vi "UDP Refresh Specific Channel and Tags.vi"(8 "error in (no error)":errorcluster, 11 "node References":T1) -> (0 "error out":errorcluster, 1 "Mapped Tag Name":string, 2 "Channel Exists?":bool, 3 "node References out":T1, 4 "tags available for mapping":refnum<class "tag descriptor.lvclass">[](array[class]))   [LabVIEW 2015, in "E2E Tag Exchange editor node.lvclass"]
uses:
  E2E Tag Exchange editor node.lvclass
  object references.ctl
  <vilib>/NI/DCAF/Tag Editor Core/Configuration Editor/Classes/Engine Parent/Engine Parent Editor Node.lvclass
  <vilib>/NI/Tag Bus/tag/tag descriptor.lvclass
  <vilib>/NI/Tag Bus Module Framework/channel/TBM channel.lvclass
  <vilib>/NI/Tag Bus/tag/tag descriptor.lvclass/tag descriptor.ctl
  <vilib>/NI/Module Execution Interface/Engine Configuration/engine configuration.lvclass
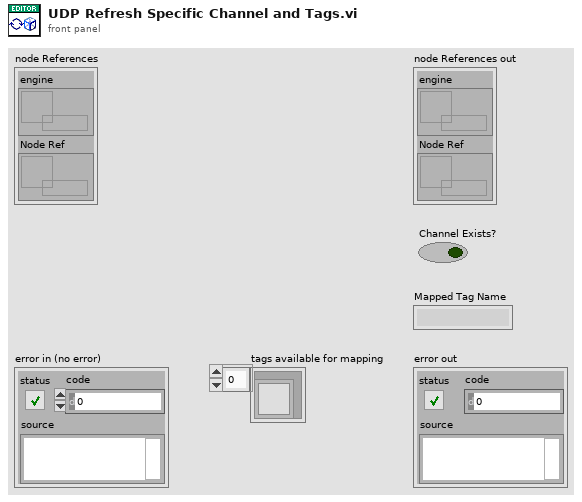
[diagram p1: front panel]
types:
  T1 = typedef "E2E Tag Exchange editor node.lvclass/object references.ctl" = cluster{"engine":refnum<data-value>, "Node Ref":refnum<data-value>}
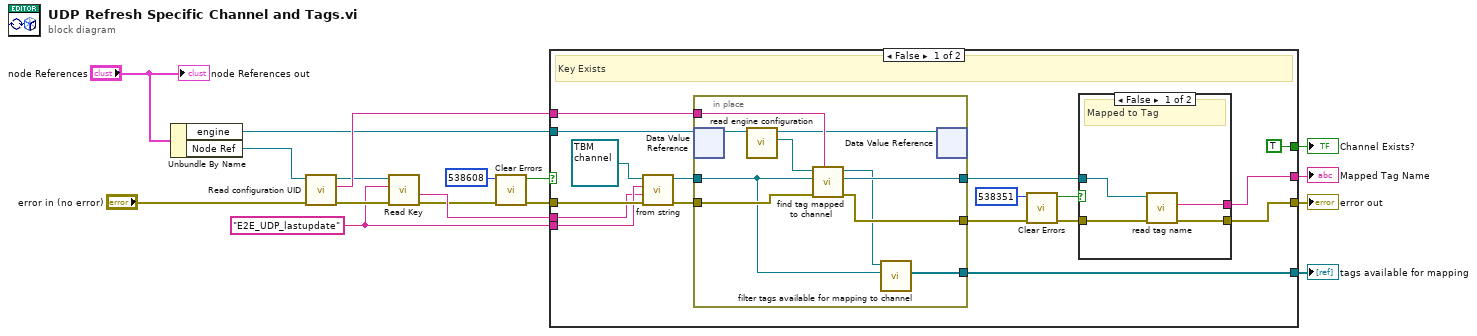
[diagram p0: block diagram]
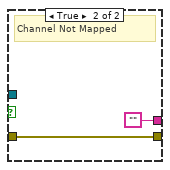
[diagram p2: hidden frame]
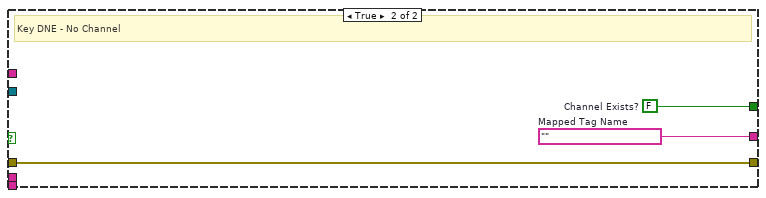
[diagram p3: hidden frame]
diagram:
  w8 = "E2E_UDP_lastupdate" ("Key")
  n1 = Unbundle By Name("node References") -> ("engine"=w10:refnum<data-value>, "Node Ref"=w14:refnum<data-value>)
  n2 = call "Read configuration UID.vi"("error in (no error)"="error in (no error)", "E2E editor node in"=w14) -> ("error out"=w12:errorcluster, "Module UID"=w13:string, "E2E editor node out"=w11:refnum<data-value>)  [unwired: 7 in]
  n3 = call "Read Key.vi"("error in (no error)"=w12, "Key"=w8, "E2E editor node in"=w11) -> ("error out"=w4:errorcluster, "Value"=w9:string)  [unwired: 6 in, 1 out]
  n4 = call <vilib>:"Clear Errors.vi"("error in (no error)"=w4, "specific error code to clear (0: all)"=538608 ("error code (0)")) -> ("error out"=w7:errorcluster, "specific error cleared?"=w6:bool)  [unwired: 4 in]
  n5 = case shown="False" w6 {
    tunnel: w7 -> [w34 w53]
    tunnel: w8 -> [w33 _]
    tunnel: w9 -> [w32 _]
    tunnel: w10 -> [w30 _]
    tunnel: w13 -> [w29 _]
    tunnel: [w21 w53] -> w2
    tunnel: [w20 w52] -> w16
    tunnel: [TRUE ("Channel Exists?") w51] -> w15
    tunnel: [w18 _] -> w1
    frame False {
      # "Key Exists"
      n6 = call-dynamic "from string.vi"("error in"=w34, "channel data"=w32, "identifier"=w33, "channel in"=refnum<class "TBM channel.lvclass"> refnum) -> ("error out"=w27:errorcluster, "channel out"=w28:refnum<class "TBM channel.lvclass">)  [unwired: 6 in]
      n7 = in-place {
        in-place-border: w29 -> [w48]
        in-place-border: w28 -> [w42]
        in-place-border: w27 -> [w47]
        in-place-border: [w45] -> w26
        in-place-border: [w44] -> w22
        in-place-border: [w41] -> w18
        n8 = in-place-dvr #1(w30) -> (w50:refnum<class "Engine Parent Editor Node.lvclass">)  [unwired: 1 out]
        n9 = call <vilib>:"read engine configuration.vi"("Engine Parent Editor Node in"=w50) -> ("engine configuration"=w49:refnum<class "engine configuration.lvclass">, "Engine Parent Editor Node out"=w46:refnum<class "Engine Parent Editor Node.lvclass">)  [unwired: 8 in, 1 out]
        n10 = call <vilib>:"find tag mapped to channel.vi"("owner"=w48, "error in"=w47, "channel"=w42, "engine configuration in"=w49) -> ("error out"=w45:errorcluster, "tag"=w44:refnum<class "tag descriptor.lvclass">, "engine configuration out"=w43:refnum<class "engine configuration.lvclass">)  [unwired: 5 in]
        n11 = call-dynamic "filter tags available for mapping to channel.vi"("channel to map to"=w42, "engine configuration in"=w43) -> ("filtered tags"=w41:refnum<class "tag descriptor.lvclass">[])  [unwired: 8 in, 1 out]
        n12 = in-place-dvr #1(w46) -> ()  [unwired: 2 out]
      }
      n13 = call <vilib>:"Clear Errors.vi"("error in (no error)"=w26, "specific error code to clear (0: all)"=538351) -> ("error out"=w23:errorcluster, "specific error cleared?"=w24:bool)  [unwired: 4 in]
      n14 = case shown="False" w24 {
        tunnel: w23 -> [w38 w40]
        tunnel: w22 -> [w37 _]
        tunnel: [w36 ""] -> w20
        tunnel: [w35 w40] -> w21
        frame False {
          # "Mapped to Tag"
          n15 = call <vilib>:"read tag name.vi"("error in"=w38, "system tag in"=w37) -> ("error out"=w35:errorcluster, "name"=w36:string)  [unwired: 7 in, 1 out]
        }
        frame True {
          # "Channel Not Mapped"
        }
      }
    }
    frame True {
      w51 = FALSE  # Channel Exists?
      w52 = ""  # Mapped Tag Name
      # "Key DNE - No Channel"
    }
  }
  "Mapped Tag Name" <- w16
  "Channel Exists?" <- w15
  "error out" <- w2
  "tags available for mapping" <- w1
  "node References out" <- "node References"
